vi "Pulse once per interval.vi"(1 "Time (ms)":u32) -> (0 "Boolean":bool)   [LabVIEW 2019]
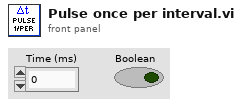
[diagram p1: front panel]
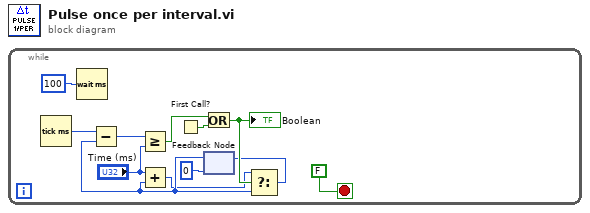
[diagram p0: block diagram]
diagram:
  n1 = while {
    stop <- FALSE stop-if-true
    n2 = Tick Count (ms)() -> (millisecond timer value=w4:u32)
    n3 = Wait (ms)(milliseconds to wait=u32 100) -> ()  [unwired: 1 out]
    n4 = First Call?() -> (First Call?: T/F=w3:bool)
    n5 = feedback #1(u32 0 ("y")) -> (w9:u32)
    n6 = Subtract(x=w4, y=w9) -> (x-y=w6:u32)
    n7 = Greater Or Equal?(x=w6, y="Time (ms)") -> (x >= y?=w5:bool)
    n8 = Add(x="Time (ms)", y=w9) -> (x+y=w8:u32)
    n9 = Or(x=w5, y=w3) -> (x .or. y?=w10:bool)
    "Boolean" <- w10
    n10 = Select(t=w8, s=w10, f=w9) -> (s? t:f=w1:u32)
    n11 = feedback-in #1(w1) -> ()
  }
